vi "parseUPnPXML.vi"(1 "XML upnp JiL":string="<root xmlns=\"urn:schemas-upnp-org:device-1-0\">\n  <specVersion>\n    <major>1</major>\n    <minor>0</minor>\n  </specVersion>\n  <device>\n    <deviceType>urn:schemas-upnp-org:device:JIL:1</deviceType>\n    <friendlyName>JIL server</friendlyName>\n    <manufacturer>UNED</manufacturer>\n    <manufacturerURL>http://www.dia.uned.es</manufacturerURL>\n    <modelDescription>Smart device for remote experimentation</modelDescription>\n    <modelName>JIL</modelName>\n    <modelNumber>1.0</modelNumber>\n    <modelURL>http:lab.dia.uned.espersonalweb</modelURL>\n    <serialNumber>1234567890</serialNumber>\n    <UDN>uuid:jilserverSmartDevice</UDN>\n    <UPC>123456789012</UPC>\n    <serviceList>\n      <service>\n        <serviceType>urn:schemas-upnp-org:service:switchOn:1</serviceType>\n        <serviceId>urn:upnp-org:serviceId:switchOn</serviceId>\n        <SCPDURL>URL to service description</SCPDURL>\n        <controlURL>URL for control</controlURL>\n        <eventSubURL>URL for eventing</eventSubURL>\n      </service>\n      <service>\n        <serviceType>urn:schemas-upnp-org:service:switchOff:1</serviceType>\n        <serviceId>urn:upnp-org:serviceId:switchOff</serviceId>\n        <SCPDURL>URL to service description</SCPDURL>\n        <controlURL>URL for control</controlURL>\n        <eventSubURL>URL for eventing</eventSubURL>\n      </service>\n    </serviceList>\n    <presentationURL>http:lab.dia.uned.espersonalweb</presentationURL>\n  </device>\n</root>") -> (0 "root":T1)   [LabVIEW 2010]
uses:
  <vilib>/xml/Close Reference(Node).vi
  <vilib>/xml/Close Reference(NdList).vi
  <vilib>/xml/NI_XML.lvlib
  Program Files/National Instruments/LabVIEW 2010/resource/objmgr/DOMUserDefRef.rc
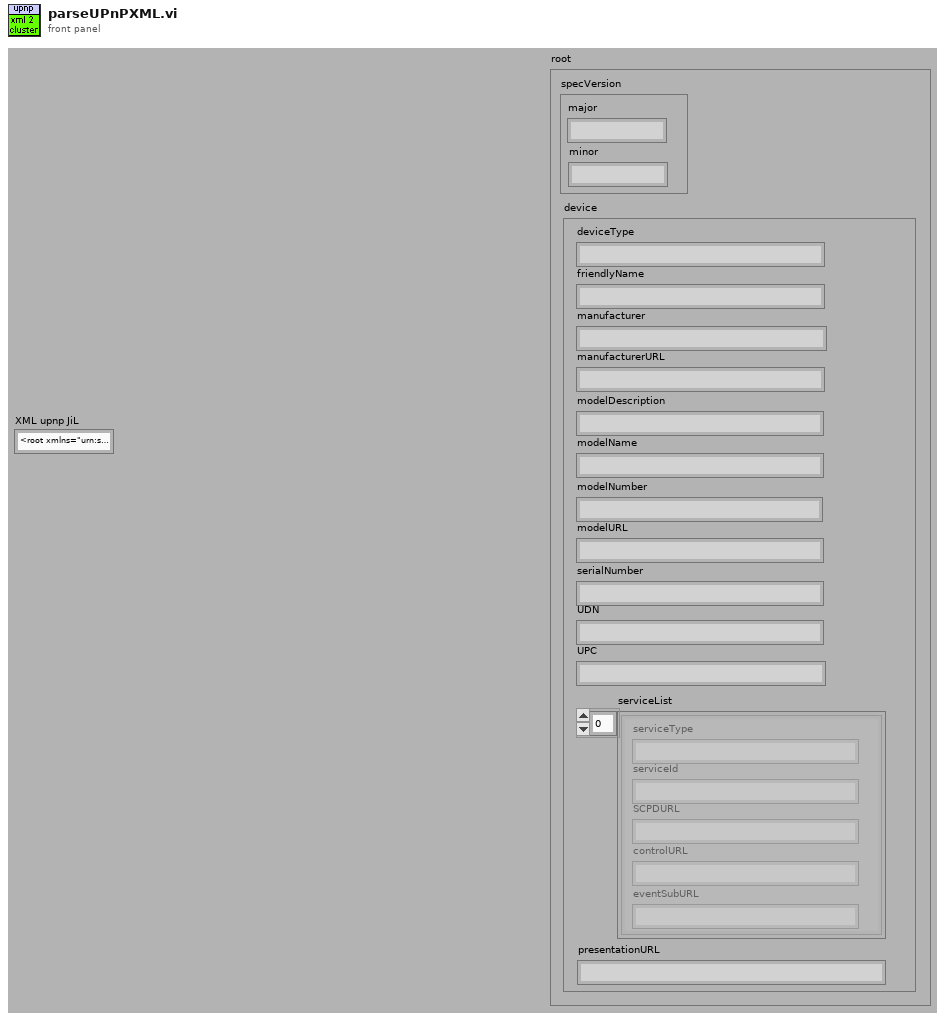
[diagram p1: front panel]
types:
  T1 = cluster{"specVersion":cluster{"major":string, "minor":string}, "device":cluster{"deviceType":string, "friendlyName":string, "manufacturer":string, "manufacturerURL":string, "modelDescription":string, "modelName":string, "modelNumber":string, "modelURL":string, "serialNumber":string, "UDN":string, "UPC":string, "serviceList":cluster{"serviceType":string, "serviceId":string, "SCPDURL":string, "controlURL":string, "eventSubURL":string}[], "presentationURL":string}}
  T2 = cluster{"deviceType":string, "friendlyName":string, "manufacturer":string, "manufacturerURL":string, "modelDescription":string, "modelName":string, "modelNumber":string, "modelURL":string, "serialNumber":string, "UDN":string, "UPC":string, "serviceList":cluster{"serviceType":string, "serviceId":string, "SCPDURL":string, "controlURL":string, "eventSubURL":string}[], "presentationURL":string}
  T3 = cluster{"serviceType":string, "serviceId":string, "SCPDURL":string, "controlURL":string, "eventSubURL":string}
  T4 = cluster{"serviceType":string, "serviceId":string, "SCPDURL":string, "controlURL":string, "eventSubURL":string}[]
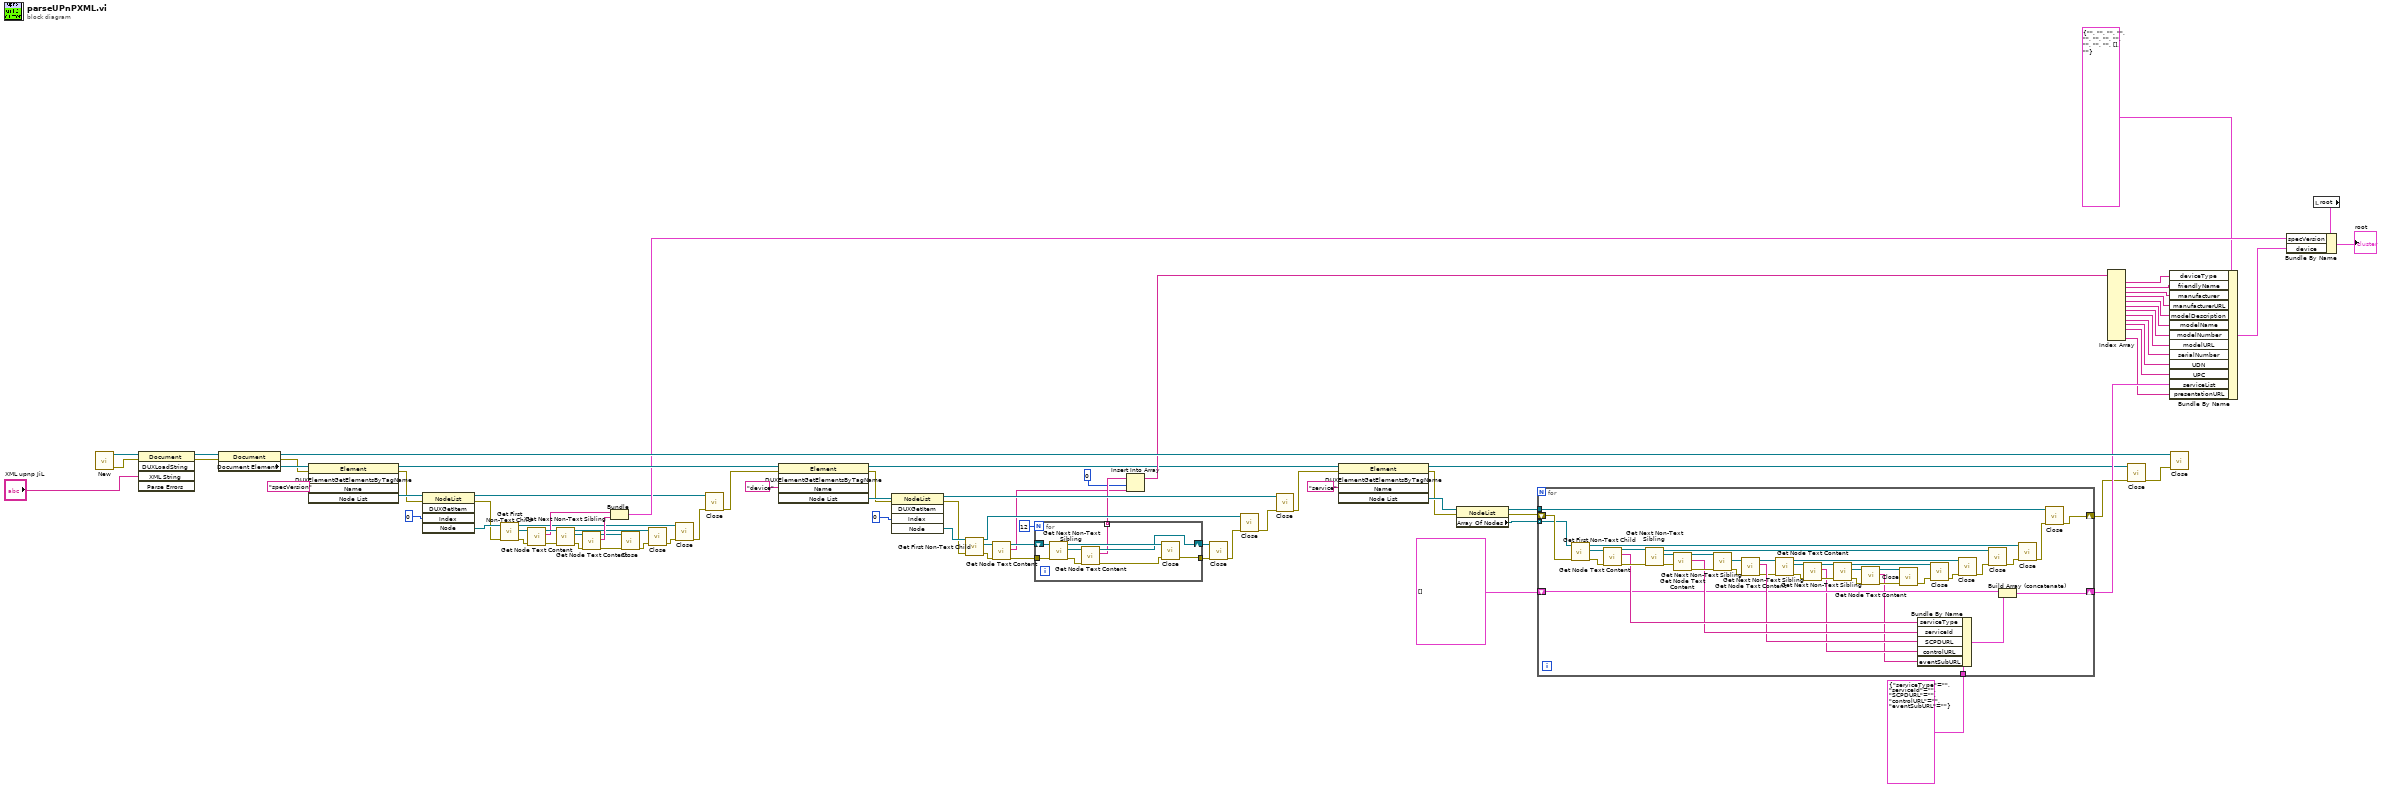
[diagram p0: block diagram]
diagram:
  n1 = call <vilib>:"New.vi"() -> ("error out"=w83:errorcluster, "DOM document out"=w84:refnum<k20>)  [unwired: 1 in, 7 out]
  n2 = invoke class="Document" method="DUXLoadString"(reference=w84, error in=w83, "XML String"="XML upnp JiL") -> (reference out=w82:refnum<k20>, error out=w81:errorcluster)  [unwired: 2 in, 3 out]
  n3 = property class="Document"(reference=w82, error in=w81) -> (reference out=w76:refnum<k20>, error out=w79:errorcluster, "Document Element"=w80:refnum<k20>)
  n4 = invoke class="Element" method="DUXElementGetElementsByTagName"(reference=w80, error in=w79, "Name"="specVersion" ("Tag Name")) -> (reference out=w77:refnum<k20>, error out=w48:errorcluster, "Node List"=w74:refnum<k20>)  [unwired: 2 in, 2 out]
  n5 = invoke class="NodeList" method="DUXGetItem"(reference=w74, error in=w48, "Index"=0) -> (reference out=w55:refnum<k20>, error out=w47:errorcluster, "Node"=w72:refnum<k20>)  [unwired: 2 in, 2 out]
  n6 = call <vilib>:"Get First Non-Text Child.vi"("error in (no error)"=w47, "node in"=w72) -> ("error out"=w70:errorcluster, "child node"=w71:refnum<k20>, "node out"=w57:refnum<k20>)  [unwired: 7 out]
  n7 = call <vilib>:"Get Node Text Content.vi"("error in (no error)"=w70, "node in"=w71) -> ("error out"=w67:errorcluster, "node text"=w65:string, "node out"=w69:refnum<k20>)  [unwired: 7 out]
  n8 = call <vilib>:"Get Next Non-Text Sibling.vi"("error in (no error)"=w67, "node in"=w69) -> ("error out"=w62:errorcluster, "sibling node"=w68:refnum<k20>, "node out"=w61:refnum<k20>)  [unwired: 7 out]
  n9 = call <vilib>:"Get Node Text Content.vi"("error in (no error)"=w62, "node in"=w68) -> ("error out"=w59:errorcluster, "node text"=w64:string, "node out"=w60:refnum<k20>)  [unwired: 7 out]
  n10 = Bundle("node text"=w65, "node text"=w64) -> (w63:cluster{"node text":string, "node text":string})  [unwired: 1 out]
  n11 = call-poly <vilib>:"Close.vi"("error in (no error)"=w59, "node"=w60) -> ("error out"=w58:errorcluster)  [unwired: 7 out]
  n12 = call-poly <vilib>:"Close.vi"("error in (no error)"=w58, "node"=w61) -> ("error out"=w56:errorcluster)  [unwired: 7 out]
  n13 = call-poly <vilib>:"Close.vi"("error in (no error)"=w56, "node"=w57) -> ("error out"=w54:errorcluster)  [unwired: 7 out]
  n14 = call-poly <vilib>:"Close.vi"("error in (no error)"=w54, "node list"=w55) -> ("error out"=w53:errorcluster)  [unwired: 7 out]
  n15 = invoke class="Element" method="DUXElementGetElementsByTagName"(reference=w77, error in=w53, "Name"="device" ("Tag Name")) -> (reference out=w17:refnum<k20>, error out=w49:errorcluster, "Node List"=w50:refnum<k20>)  [unwired: 2 in, 2 out]
  n16 = invoke class="NodeList" method="DUXGetItem"(reference=w50, error in=w49, "Index"=0) -> (reference out=w38:refnum<k20>, error out=w43:errorcluster, "Node"=w44:refnum<k20>)  [unwired: 2 in, 2 out]
  n17 = call <vilib>:"Get First Non-Text Child.vi"("error in (no error)"=w43, "node in"=w44) -> ("error out"=w45:errorcluster, "child node"=w46:refnum<k20>, "node out"=w40:refnum<k20>)  [unwired: 7 out]
  n18 = call <vilib>:"Get Node Text Content.vi"("error in (no error)"=w45, "node in"=w46) -> ("error out"=w41:errorcluster, "node text"=w34:string, "node out"=w42:refnum<k20>)  [unwired: 7 out]
  n19 = for {
    N: 12 -> [_]
    tunnel: w41 -> [w91]
    shift-right: [w87] -> w21
    shift-left: w42 -> [w93]
    tunnel: [w88] -> w20
    tunnel: [w85] -> w36 mode=indexing
    n20 = call <vilib>:"Get Next Non-Text Sibling.vi"("error in (no error)"=w91, "node in"=w93) -> ("error out"=w90:errorcluster, "sibling node"=w92:refnum<k20>, "node out"=w89:refnum<k20>)  [unwired: 7 out]
    n21 = call <vilib>:"Get Node Text Content.vi"("error in (no error)"=w90, "node in"=w92) -> ("error out"=w86:errorcluster, "node text"=w85:string, "node out"=w87:refnum<k20>)  [unwired: 7 out]
    n22 = call-poly <vilib>:"Close.vi"("error in (no error)"=w86, "node"=w89) -> ("error out"=w88:errorcluster)  [unwired: 7 out]
  }
  n23 = Insert Into Array(array=w36, index=0, new element=w34) -> (w33:string[])
  n24 = call-poly <vilib>:"Close.vi"("error in (no error)"=w20, "node"=w21) -> ("error out"=w19:errorcluster)  [unwired: 7 out]
  n25 = call-poly <vilib>:"Close.vi"("error in (no error)"=w19, "node"=w40) -> ("error out"=w37:errorcluster)  [unwired: 7 out]
  n26 = call-poly <vilib>:"Close.vi"("error in (no error)"=w37, "node list"=w38) -> ("error out"=w16:errorcluster)  [unwired: 7 out]
  n27 = invoke class="Element" method="DUXElementGetElementsByTagName"(reference=w17, error in=w16, "Name"="service" ("Tag Name")) -> (reference out=w4:refnum<k20>, error out=w14:errorcluster, "Node List"=w15:refnum<k20>)  [unwired: 2 in, 2 out]
  n28 = property class="NodeList"(reference=w15, error in=w14) -> (reference out=w11:refnum<k20>, error out=w12:errorcluster, "Array Of Nodes"=w13:refnum<k20>[])
  n29 = for {
    tunnel: w13 -> [w110] mode=indexing
    tunnel: w11 -> [w121]
    shift-right: [w113] -> w8
    shift-left: T4 [] -> [w115]
    shift-right: [w120] -> w3
    shift-left: w12 -> [w112]
    tunnel: T3 {"serviceType"="", "serviceId"="", "SCPDURL"="", "controlURL"="", "eventSubURL"=""} -> [w119]
    n30 = call <vilib>:"Get First Non-Text Child.vi"("error in (no error)"=w112, "node in"=w110) -> ("error out"=w134:errorcluster, "child node"=w135:refnum<k20>, "node out"=w127:refnum<k20>)  [unwired: 7 out]
    n31 = call <vilib>:"Get Node Text Content.vi"("error in (no error)"=w134, "node in"=w135) -> ("error out"=w130:errorcluster, "node text"=w118:string, "node out"=w131:refnum<k20>)  [unwired: 7 out]
    n32 = call <vilib>:"Get Next Non-Text Sibling.vi"("error in (no error)"=w130, "node in"=w131) -> ("error out"=w133:errorcluster, "sibling node"=w132:refnum<k20>, "node out"=w129:refnum<k20>)  [unwired: 7 out]
    n33 = call <vilib>:"Get Node Text Content.vi"("error in (no error)"=w133, "node in"=w132) -> ("error out"=w124:errorcluster, "node text"=w117:string, "node out"=w125:refnum<k20>)  [unwired: 7 out]
    n34 = call <vilib>:"Get Next Non-Text Sibling.vi"("error in (no error)"=w124, "node in"=w125) -> ("error out"=w123:errorcluster, "sibling node"=w122:refnum<k20>)  [unwired: 8 out]
    n35 = call <vilib>:"Get Node Text Content.vi"("error in (no error)"=w123, "node in"=w122) -> ("error out"=w104:errorcluster, "node text"=w116:string, "node out"=w107:refnum<k20>)  [unwired: 7 out]
    n36 = call <vilib>:"Get Next Non-Text Sibling.vi"("error in (no error)"=w104, "node in"=w107) -> ("error out"=w109:errorcluster, "sibling node"=w95:refnum<k20>, "node out"=w99:refnum<k20>)  [unwired: 7 out]
    n37 = call <vilib>:"Get Node Text Content.vi"("error in (no error)"=w109, "node in"=w95) -> ("error out"=w105:errorcluster, "node text"=w97:string, "node out"=w106:refnum<k20>)  [unwired: 7 out]
    n38 = call <vilib>:"Get Next Non-Text Sibling.vi"("error in (no error)"=w105, "node in"=w106) -> ("error out"=w108:errorcluster, "sibling node"=w94:refnum<k20>, "node out"=w100:refnum<k20>)  [unwired: 7 out]
    n39 = call <vilib>:"Get Node Text Content.vi"("error in (no error)"=w108, "node in"=w94) -> ("error out"=w101:errorcluster, "node text"=w96:string, "node out"=w102:refnum<k20>)  [unwired: 7 out]
    n40 = call-poly <vilib>:"Close.vi"("error in (no error)"=w101, "node"=w102) -> ("error out"=w103:errorcluster)  [unwired: 7 out]
    n41 = Bundle By Name(cluster=w119, "serviceType"=w118, "serviceId"=w117, "SCPDURL"=w116, "controlURL"=w97, "eventSubURL"=w96) -> (w114:T3)
    n42 = call-poly <vilib>:"Close.vi"("error in (no error)"=w103, "node"=w100) -> ("error out"=w98:errorcluster)  [unwired: 7 out]
    n43 = call-poly <vilib>:"Close.vi"("error in (no error)"=w98, "node"=w99) -> ("error out"=w128:errorcluster)  [unwired: 7 out]
    n44 = call-poly <vilib>:"Close.vi"("error in (no error)"=w128, "node"=w129) -> ("error out"=w126:errorcluster)  [unwired: 7 out]
    n45 = Build Array (concatenate)(w115, w114) -> (w113:T4)
    n46 = call-poly <vilib>:"Close.vi"("error in (no error)"=w126, "node"=w127) -> ("error out"=w111:errorcluster)  [unwired: 7 out]
    n47 = call-poly <vilib>:"Close.vi"("error in (no error)"=w111, "node list"=w121) -> ("error out"=w120:errorcluster)  [unwired: 7 out]
  }
  n48 = Index Array(array=w33) -> (element #1=w32:string, element #2=w31:string, element #3=w30:string, element #4=w29:string, element #5=w28:string, element #6=w27:string, element #7=w26:string, element #8=w25:string, element #9=w24:string, element #10=w23:string, element #11=w22:string, element #13=w2:string)  [unwired: 13 in, 1 out]
  n49 = call-poly <vilib>:"Close.vi"("error in (no error)"=w3, "node"=w4) -> ("error out"=w52:errorcluster)  [unwired: 7 out]
  n50 = Bundle By Name(cluster=T2 {"deviceType"="", "friendlyName"="", "manufacturer"="", "manufacturerURL"="", "modelDescription"="", "modelName"="", "modelNumber"="", "modelURL"="", "serialNumber"="", "UDN"="", "UPC"="", "serviceList"=[], "presentationURL"=""} ("device"), "deviceType"=w32, "friendlyName"=w31, "manufacturer"=w30, "manufacturerURL"=w29, "modelDescription"=w28, "modelName"=w27, "modelNumber"=w26, "modelURL"=w25, "serialNumber"=w24, "UDN"=w23, "UPC"=w22, "serviceList"=w8, "presentationURL"=w2) -> (w6:T2)
  n51 = call-poly <vilib>:"Close.vi"("error in (no error)"=w52, "node"=w76) -> ()  [unwired: 8 out]
  n52 = local read "root"() -> (w66:T1)
  n53 = Bundle By Name(cluster=w66, "specVersion"=w63, "device"=w6) -> (→"root":T1)
